vi "MT Compensate Sample Clock Frequency Error (FSK).vi"(0 "input complex waveform":cluster{"t0":dbl, "dt":dbl, "Y":cdb[]}={"t0"=0.0, "dt"=1.0416666666666667e-06, "Y"=array[11712 elements]}, 5 "samples per symbol":i32, 7 "matched filter coefficients":dbl[](array[numeric]) format="%.2f", 9 "clock phase computation window (symbols)":i32=64, 11 "error in (no error)":errorcluster) -> (4 "output complex waveform":T1 {"Y" format="%.3f"; "dt" format="%^.2e"; "t0" format="%.4f"}, 6 "sample clock frequency error (ppm)":dbl, 15 "error out":errorcluster)   [LabVIEW 2020, in "niDMT.lvlib"]
doc: "This polymorphic instance corrects the sample clock frequency offset before calling the MT Demodulate FSK VI."
uses:
  <vilib>/addons/Modulation/niDMT.lvlib
  <vilib>/addons/Modulation/Analog/controls/Complex Data Waveform.ctl
  <vilib>/Analysis/baseanly.llb/Mean (DBL).vi
  <vilib>/addons/Modulation/Analog/support/Validators/mod_WFErrorHandler.vi
  <vilib>/addons/Modulation/Analog/support/Validators/mod_Fractional Resample Validate.vi
  <vilib>/addons/Modulation/Analog/support/Validators/mod_Check Flush State.vi
  <vilib>/addons/Modulation/Analog/support/mod_FractionalResampler.vi
  <vilib>/addons/Modulation/Analog/support/mod_Integer Rate Interpolation.vi
  <vilib>/addons/Modulation/Analog/support/mod_Set Error Source.vi
  <vilib>/addons/Modulation/Analog/support/mod_PerformResampling.vi
  <vilib>/addons/Modulation/Digital/General/MT Apply Matched Filter (FSK).vi
  <vilib>/Utility/error.llb/Error Cluster From Error Code.vi
  <vilib>/addons/Modulation/Analog/support/mod_Resampling Factors.vi
  <vilib>/addons/Modulation/Analog/support/mod_ResamplingFilter.vi
  <vilib>/addons/Modulation/Analog/support/mod_Generate Integer Interpolation Filter.vi
  <vilib>/addons/Modulation/niAMT.lvlib
  <vilib>/Analysis/NI_AALPro.lvlib
  <vilib>/Analysis/NI_AALBase.lvlib
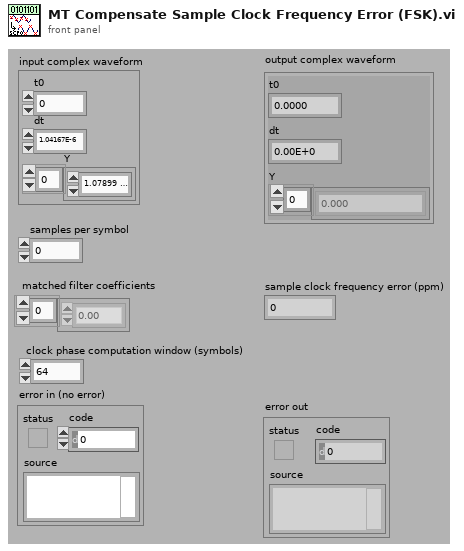
[diagram p1: front panel]
types:
  T1 = typedef "niAMT.lvlib/Complex Data Waveform.ctl" = cluster{"t0":dbl, "dt":dbl, "Y":cdb[]}
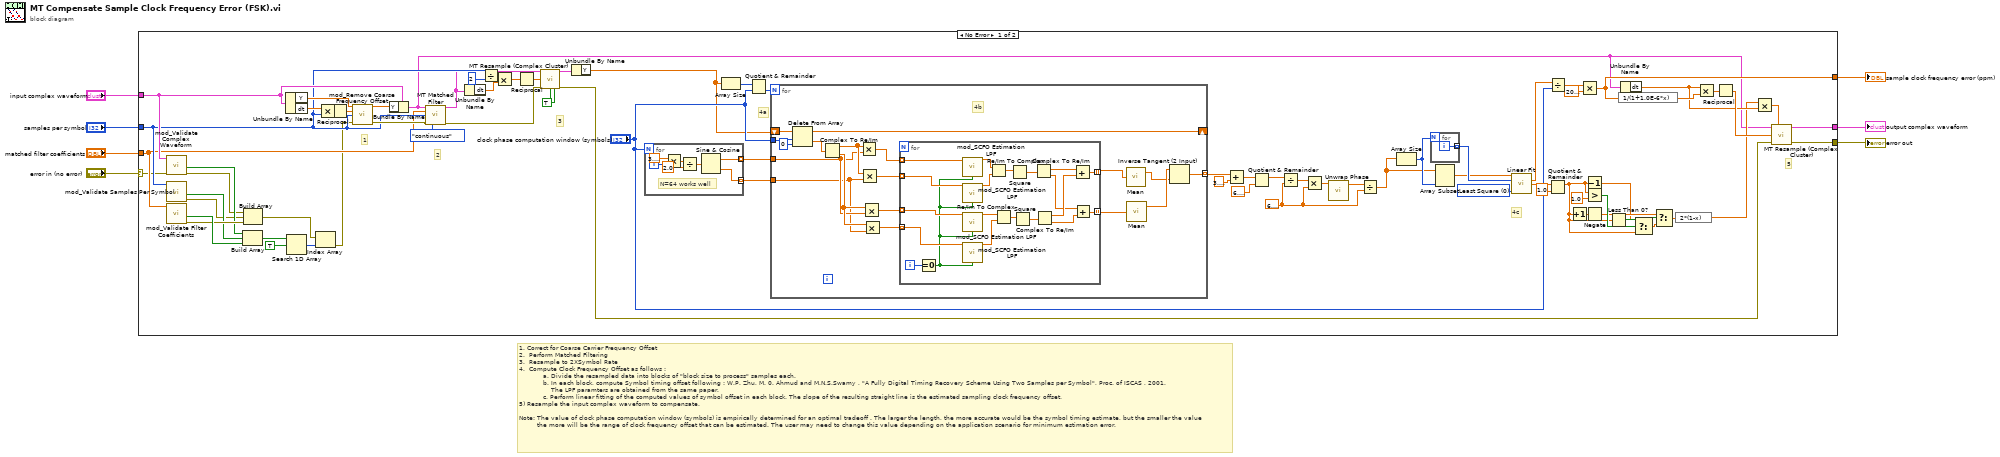
[diagram p0: block diagram]
diagram:
  # "1.\tCorrect for Coarse Carrier Frequency Offset\n2.\t Perform Matched Filtering\n3. \tResample to 2XSymbol Rate\n4. \tCompute Clock Frequency Offset as follows : \n            a.\tDivide the resampled data into blocks of \"block size to process\" samples each. \n            b.\tIn each block, compute Symbol timing offset following : W.P. Zhu, M. 0. Ahmud and M.N.S.Swamy , \"A Fully Digital Timing Recovery Scheme Using Two Samples per Symbol\", Proc. of ISCAS , 2001. \n                The LPF paramters are obtained from the same paper. \n            c.\tPerform linear fitting of the computed values of symbol offset in each block. The slope of the resulting straight line is the estimated sampling clock frequency offset. \n5)\tResample the input complex waveform to compensate.\n\nNote: The value of clock phase computation window (symbols) is empirically determined for an optimal tradeoff . The larger the length, the more accurate would be the symbol timing estimate, but the smaller the value \n         the more will be the range of clock frequency offset that can be estimated. The user may need to change this value depending on the application scenario for minimum estimation error."
  n1 = case shown="No Error" "error in (no error)" {
    selector: "error in (no error)" -> [w11 w130]
    tunnel: "input complex waveform" -> [w14 _]
    tunnel: [w63 _] -> w6
    tunnel: [w35 _] -> w5
    tunnel: "samples per symbol" -> [w13 _]
    tunnel: "matched filter coefficients" -> [w12 _]
    tunnel: [w25 w130] -> w2
    frame No Error {
      w68 = u16 0 items=["Least Square", "Least Absolute Residual", "Bisquare"] ("method")
      w70 = 6.283185307179586
      w44 = TRUE ("reset? (T)")
      # "5"
      # "4c"
      # "4a"
      # "3"
      # "2"
      # "1"
      n2 = call <vilib>:"mod_Validate Complex Waveform.vi"("error in (no error)"=w11, "input complex waveform"=w14) -> ("error out"=w20:errorcluster, "error?"=w22:bool)  [unwired: 8 out]
      n3 = call <vilib>:"mod_Validate Samples Per Symbol.vi"("Samples Per Symbol"=w13) -> ("error out"=w19:errorcluster, "error?"=w21:bool)  [unwired: 9 out]
      n4 = call <vilib>:"mod_Validate Filter Coefficients.vi"("Filter Coefficients"=w12) -> ("error out"=w23:errorcluster, "error?"=w24:bool)  [unwired: 9 out]
      n5 = Build Array(w22, w21, w24) -> (w17:bool[])
      n6 = Build Array(w20, w19, w23) -> (w18:errorcluster[])
      n7 = Unbundle By Name(w14) -> ("Y"=w83:cdb[], "dt"=w82:dbl)
      n8 = Search 1D Array(1D array=w17, element=TRUE) -> (index of element=w15:i32)  [unwired: 1 out]
      n9 = Index Array(array=w18, index=w15) -> (element=w10:errorcluster)
      n10 = Multiply(x=w82, y=w13) -> (x*y=w81:dbl)
      n11 = Reciprocal(x=w81) -> (1/x=w80:dbl)
      n12 = call <vilib>:"mod_Remove Coarse Frequency Offset.vi"("Signal In"=w83, "Symbol Rate, Hz"=w80, "Samples Per Symbol (16)"=w13, "error in (no error)"=w10) -> ("Signal Out"=w79:cdb[], "error out"=w28:errorcluster)  [unwired: 1 in, 9 out]
      n13 = Bundle By Name(cluster=w14, "Y"=w79) -> (w9:cluster{"t0":dbl, "dt":dbl, "Y":cdb[]})
      n14 = call-poly <vilib>:"MT Matched Filter.vi"("input complex waveform"=w9, "matched filter coefficients"=w12, "samples per symbol (16)"=w13, "error in (no error)"=w28, "symbol phase continuity"=enum16{"continuous", "discontinuous"}."continuous") -> ("output phase waveform"=w8:cluster{"t0":dbl, "dt":dbl, "Y":dbl[]}, "error out"=w27:errorcluster)  [unwired: 2 in, 7 out]
      n15 = Unbundle By Name(w8) -> ("dt"=w43:dbl)
      n16 = Divide(x=w13, y=2) -> (x/y=w46:dbl)
      n17 = Multiply(x=w46, y=w43) -> (x*y=w42:dbl)
      n18 = Reciprocal(x=w42) -> (1/x=w45:dbl)
      n19 = call <vilib>:"MT Resample (Complex Cluster).vi"("input complex waveform"=w8, "desired sample rate (Hz)"=w45, "error in (no error)"=w27, "reset? (T)"=w44, "flush buffers? (F)"=w44) -> ("output complex waveform"=w36:T1, "error out"=w26:errorcluster)  [unwired: 1 in, 8 out]
      n20 = Unbundle By Name(w36) -> ("Y"=w32:cdb[])
      n21 = for {
        N: "clock phase computation window (symbols)" -> [_]
        tunnel: [w124] -> w76 mode=indexing
        tunnel: [w123] -> w48 mode=indexing
        i -> [w128]
        # "N=64 works well"
        n22 = Multiply(x=3.141592653589793, y=w128) -> (x*y=w127:dbl)
        n23 = Divide(x=w127, y=2.0) -> (x/y=w125:dbl)
        n24 = Sine & Cosine(0:w125) -> (1:w124:dbl, 2:w123:dbl)
      }
      n25 = Array Size(array=w32) -> (size(s)=w78:i32)
      n26 = Quotient & Remainder(x=w78, y="clock phase computation window (symbols)") -> (floor(x/y)=w77:i32)  [unwired: 1 out]
      n27 = for {
        N: w77 -> [_]
        shift-right: [w99] -> _
        shift-left: w32 -> [w102]
        tunnel: "clock phase computation window (symbols)" -> [w101]
        tunnel: w76 -> [w96]
        tunnel: w48 -> [w95]
        tunnel: [w86] -> w75 mode=indexing
        # "4b"
        n28 = Delete From Array(array=w102, length=w101, index=0) -> (deleted portion=w85:cdb[], array with subset deleted=w99:cdb[])
        n29 = Complex To Re/Im(x + iy=w85) -> (x=w98:dbl[], y=w97:dbl[])
        n30 = Multiply(x=w98, y=w96) -> (x*y=w94:dbl[])
        n31 = Multiply(x=w98, y=w95) -> (x*y=w93:dbl[])
        n32 = Multiply(x=w97, y=w96) -> (x*y=w92:dbl[])
        n33 = Multiply(x=w97, y=w95) -> (x*y=w91:dbl[])
        n34 = for {
          tunnel: w94 -> [w122] mode=indexing
          tunnel: w93 -> [w120] mode=indexing
          tunnel: w92 -> [w119] mode=indexing
          tunnel: w91 -> [w118] mode=indexing
          tunnel: [w104] -> w90 mode=indexing
          tunnel: [w103] -> w89 mode=indexing
          i -> [w121]
          n35 = Equal To 0?(x=w121) -> (x = 0?=w117:bool)
          n36 = call <vilib>:"mod_SCFO Estimation LPF.vi"("x[n]"=w122, "reset"=w117) -> ("y[n]"=w116:dbl)  [unwired: 13 out]
          n37 = call <vilib>:"mod_SCFO Estimation LPF.vi"("x[n]"=w120, "reset"=w117) -> ("y[n]"=w115:dbl)  [unwired: 13 out]
          n38 = call <vilib>:"mod_SCFO Estimation LPF.vi"("x[n]"=w119, "reset"=w117) -> ("y[n]"=w114:dbl)  [unwired: 13 out]
          n39 = call <vilib>:"mod_SCFO Estimation LPF.vi"("x[n]"=w118, "reset"=w117) -> ("y[n]"=w113:dbl)  [unwired: 13 out]
          n40 = Re/Im To Complex(1:w115, 2:w116) -> (0:w112:cdb)
          n41 = Re/Im To Complex(1:w113, 2:w114) -> (0:w111:cdb)
          n42 = Square(x=w112) -> (x^2=w110:cdb)
          n43 = Square(x=w111) -> (x^2=w109:cdb)
          n44 = Complex To Re/Im(x + iy=w110) -> (x=w108:dbl, y=w106:dbl)
          n45 = Complex To Re/Im(x + iy=w109) -> (x=w107:dbl, y=w105:dbl)
          n46 = Add(x=w108, y=w107) -> (x+y=w104:dbl)
          n47 = Add(x=w106, y=w105) -> (x+y=w103:dbl)
        }
        n48 = call-poly <vilib>:"Mean.vi"("X"=w90) -> ("mean"=w87:dbl)  [unwired: 1 out]
        n49 = call-poly <vilib>:"Mean.vi"("X"=w89) -> ("mean"=w88:dbl)  [unwired: 1 out]
        n50 = Inverse Tangent (2 Input)(1:w87, 2:w88) -> (0:w86:dbl)
      }
      n51 = Add(x=w75, y=3.141592653589793) -> (x+y=w51:dbl[])
      n52 = Quotient & Remainder(x=w51, y=6.283185307179586) -> (x-y*floor(x/y)=w50:dbl[])  [unwired: 1 out]
      n53 = Divide(x=w50, y=w70) -> (x/y=w49:dbl[])
      n54 = Multiply(x=w49, y=w70) -> (x*y=w72:dbl[])
      n55 = call <vilib>:"Unwrap Phase.vi"("Phase"=w72) -> ("Unwrapped Phase"=w71:dbl[])  [unwired: 1 in, 9 out]
      n56 = Divide(x=w71, y=w70) -> (x/y=w66:dbl[])
      n57 = Array Size(array=w66) -> (size(s)=w69:i32)
      n58 = for {
        N: w69 -> [_]
        tunnel: [w84] -> w67 mode=indexing
        i -> [w84]
      }
      n59 = Array Subset(array=w66, length=w69) -> (w34:dbl[])  [unwired: 1 in]
      n60 = call <vilib>:"Linear Fit.vi"("Y"=w34, "X"=w67, "method"=w68) -> ("slope"=w62:dbl, "intercept"=w54:dbl)  [unwired: 3 in, 8 out]
      n61 = Divide(x=w62, y="clock phase computation window (symbols)") -> (x/y=w41:dbl)
      n62 = Quotient & Remainder(x=w54, y=1.0) -> (x-y*floor(x/y)=w53:dbl)  [unwired: 1 out]
      n63 = Increment(x=w53) -> (x+1=w60:dbl)
      n64 = Multiply(x=w41, y=2000000.0) -> (x*y=w35:dbl)
      n65 = Negate(x=w60) -> (-x=w59:dbl)
      n66 = Decrement(x=w53) -> (x-1=w56:dbl)
      n67 = Greater?(x=w53, y=1.0) -> (0:w64:bool)
      n68 = Less Than 0?(x=w53) -> (x < 0?=w61:bool)
      n69 = expression code="1/(1+1.0E-6*x)"(w35) -> (w39:dbl)
      n70 = Unbundle By Name(w9) -> ("dt"=w33:dbl)
      n71 = Select(t=w56, s=w64, f=w53) -> (s? t:f=w58:dbl)
      n72 = Select(t=w59, s=w61, f=w58) -> (s? t:f=w57:dbl)
      n73 = expression code="2*(1-x)"(w57) -> (w31:dbl)
      n74 = Multiply(x=w33, y=w39) -> (x*y=w38:dbl)
      n75 = Reciprocal(x=w38) -> (1/x=w37:dbl)
      n76 = Multiply(x=w31, y=w33) -> (x*y=w30:dbl)
      n77 = call <vilib>:"MT Resample (Complex Cluster).vi"("input complex waveform"=w9, "initial sample offset (sec)"=w30, "desired sample rate (Hz)"=w37, "error in (no error)"=w26) -> ("output complex waveform"=w63:T1, "error out"=w25:errorcluster)  [unwired: 2 in, 8 out]
    }
    frame Error {
    }
  }
  "sample clock frequency error (ppm)" <- w5
  "output complex waveform" <- w6
  "error out" <- w2
